vi "ziSetValueDemod.vi"(5 "Order (2)":i32=1 min=1, 6 "Rate (200Hz)":dbl=200.0, 7 "Time Constant (1ms)":dbl=0.001, 8 "error in":errorcluster, 9 "Signal Input Select (0)":i32, 10 "Demodulator # (0)":i32, 11 "handle in":T1 {"Handle" format="0x%08x"; "Conn" format="0x%08x"}) -> (0 "error out":errorcluster, 3 "handle out":T1 {"Handle" format="0x%08x"; "Conn" format="0x%08x"})   [LabVIEW 2009, in "Zurich Instruments LabOne.lvlib"]
doc: "Helper vi to comfortably configure a Demodulator. This vi brings a demodulator into a defined state by executing a number of setValueDouble calls."
uses:
  <instrlib>/Zurich Instruments LabOne/Zurich Instruments LabOne.lvlib
  <instrlib>/Zurich Instruments LabOne/Public/ziTypeHandle.ctl
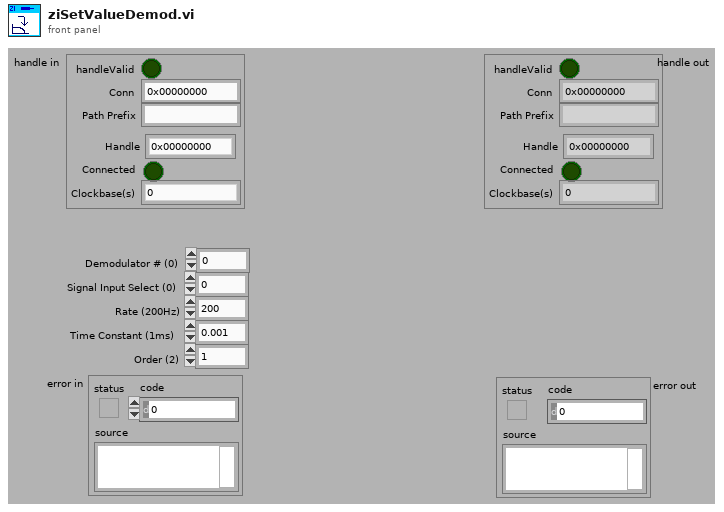
[diagram p1: front panel]
types:
  T1 = typedef "Zurich Instruments LabOne.lvlib/ziTypeHandle.ctl" = cluster{"handleValid":bool, "Conn":u64, "Path Prefix":string, "Handle":u64, "Connected":bool, "Clockbase(s)":dbl}
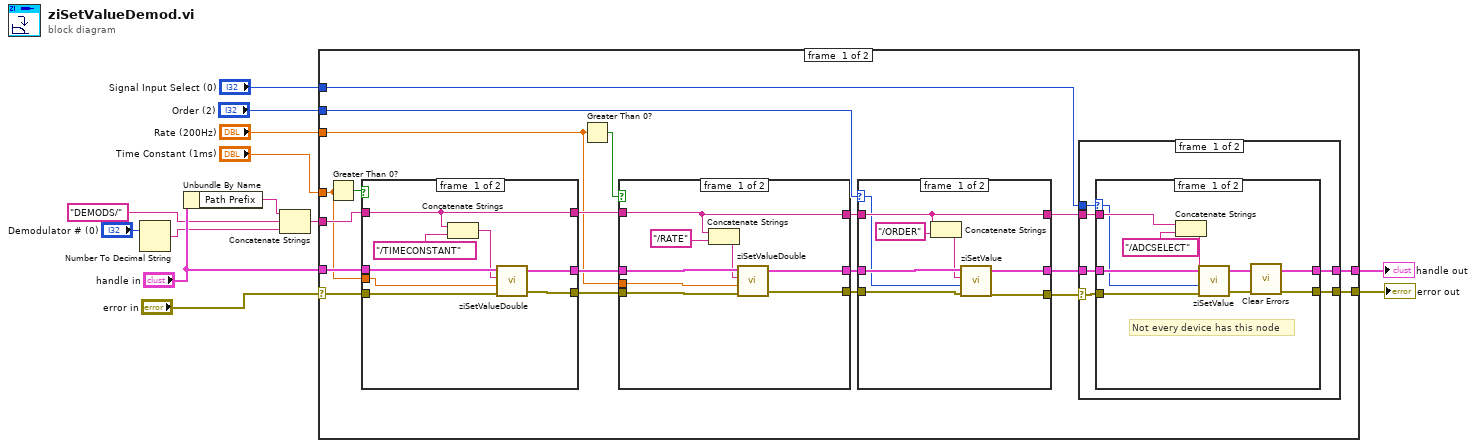
[diagram p0: block diagram]
diagram:
  n1 = Number To Decimal String(number="Demodulator # (0)") -> (decimal integer string=w1:string)  [unwired: 1 out]
  n2 = Unbundle By Name("handle in") -> ("Path Prefix"=w7:string)
  n3 = Concatenate Strings(w7, "DEMODS/", w1) -> (w5:string)
  n4 = case shown="No Error" "error in" {
    selector: "error in" -> [w16 w87]
    tunnel: "Time Constant (1ms)" -> [w15 _]
    tunnel: "Order (2)" -> [w33 _]
    tunnel: "Signal Input Select (0)" -> [w32 _]
    tunnel: [w28 w86] -> w10
    tunnel: [w25 w87] -> w9
    tunnel: "handle in" -> [w24 w86]
    tunnel: w5 -> [w20 _]
    tunnel: "Rate (200Hz)" -> [w18 _]
    frame #0 {
      n5 = Greater Than 0?(x=w15) -> (x > 0?=w14:bool)
      n6 = case shown="True" w14 {
        tunnel: w24 -> [w82 w85]
        tunnel: [w81 w85] -> w31
        tunnel: [w80 w84] -> w26
        tunnel: w16 -> [w79 w84]
        tunnel: w20 -> [w78 w83]
        tunnel: [w78 w83] -> w23
        tunnel: w15 -> [w75 _]
        frame #0 {
          n7 = Concatenate Strings(w78, "/TIMECONSTANT") -> (w76:string)
          n8 = call <instrlib>:"ziSetValueDouble.vi"("Error In"=w79, "Value"=w75, "Path"=w76, "Handle In"=w82) -> ("Error Out"=w80:errorcluster, "Handle Out"=w81:T1)  [unwired: 1 in]
        }
        frame #1 {
        }
      }
      n9 = Greater Than 0?(x=w18) -> (x > 0?=w19:bool)
      n10 = case shown="True" w19 {
        tunnel: w31 -> [w71 w74]
        tunnel: [w70 w74] -> w30
        tunnel: [w69 w73] -> w27
        tunnel: w26 -> [w68 w73]
        tunnel: w23 -> [w65 w72]
        tunnel: [w65 w72] -> w22
        tunnel: w18 -> [w64 _]
        frame #0 {
          n11 = Concatenate Strings(w65, "/RATE") -> (w66:string)
          n12 = call <instrlib>:"ziSetValueDouble.vi"("Error In"=w68, "Value"=w64, "Path"=w66, "Handle In"=w71) -> ("Error Out"=w69:errorcluster, "Handle Out"=w70:T1)  [unwired: 1 out]
        }
        frame #1 {
        }
      }
      n13 = case shown="Default" w33 {
        selector: w33 -> [w53 _]
        tunnel: w30 -> [w60 w63]
        tunnel: [w59 w63] -> w29
        tunnel: [w58 w62] -> w17
        tunnel: w27 -> [w57 w62]
        tunnel: w22 -> [w54 w61]
        tunnel: [w54 w61] -> w21
        frame #0 {
          n14 = Concatenate Strings(w54, "/ORDER") -> (w55:string)
          n15 = call-poly <instrlib>:"ziSetValue.vi"("Error In"=w57, "Value"=w53, "Path"=w55, "Handle In"=w60) -> ("Error Out"=w58:errorcluster, "Handle Out"=w59:T1)  [unwired: 1 in]
        }
        frame #1 {
        }
      }
      n16 = case shown="No Error" w17 {
        selector: w17 -> [w34 w51]
        tunnel: w32 -> [w39 _]
        tunnel: w29 -> [w38 w52]
        tunnel: [w37 w52] -> w28
        tunnel: [w36 w51] -> w25
        tunnel: w21 -> [w35 _]
        frame #0 {
          n17 = case shown="Default" w39 {
            selector: w39 -> [w41 _]
            tunnel: w38 -> [w48 w50]
            tunnel: [w47 w50] -> w37
            tunnel: w34 -> [w46 w49]
            tunnel: [w40 w49] -> w36
            tunnel: w35 -> [w44 _]
            frame #0 {
              # "Not every device has this node"
              n18 = Concatenate Strings(w44, "/ADCSELECT") -> (w43:string)
              n19 = call-poly <instrlib>:"ziSetValue.vi"("Error In"=w46, "Value"=w41, "Path"=w43, "Handle In"=w48) -> ("Error Out"=w45:errorcluster, "Handle Out"=w47:T1)  [unwired: 1 in]
              n20 = call <vilib>:"Clear Errors.vi"("error in (no error)"=w45) -> ("error out"=w40:errorcluster)  [unwired: 6 in]
            }
            frame #1 {
            }
          }
        }
        frame #1 {
        }
      }
    }
    frame #1 {
    }
  }
  "handle out" <- w10
  "error out" <- w9
